vi "Set Start Trigger (Value Change).vi"(5 "Retriggerable (F)":bool, 7 "Pre-Trigger Duration (0 s)":dbl, 8 "error in (no error)":errorcluster, 9 "Trigger Channel":string, 10 "Deadband":dbl, 11 "Data Logging Specification Ref in":T1) -> (0 "error out":errorcluster, 3 "Data Logging Specification Ref out":T1)   [LabVIEW 2020, in "NI_VS Data Logging API.lvlib"]
doc: "Specifies a trigger condition on which to start logging data. You also can specify whether to log channel data immediately preceding the trigger condition and whether logging is retriggerable, meaning the data logging session watches for subsequent occurrences of the start trigger after the first logging operation finishes. By default, logging stops after one operation.\n\nYou must manually select the polymorphic instance to use."
uses:
  <vilib>/NI VeriStand/Execution/DataLogging/NI_VS Data Logging API.lvlib
  <vilib>/NI VeriStand/Execution/DataLogging/DataLoggingSpecification Ref.ctl
  NationalInstruments.VeriStand.ClientAPI
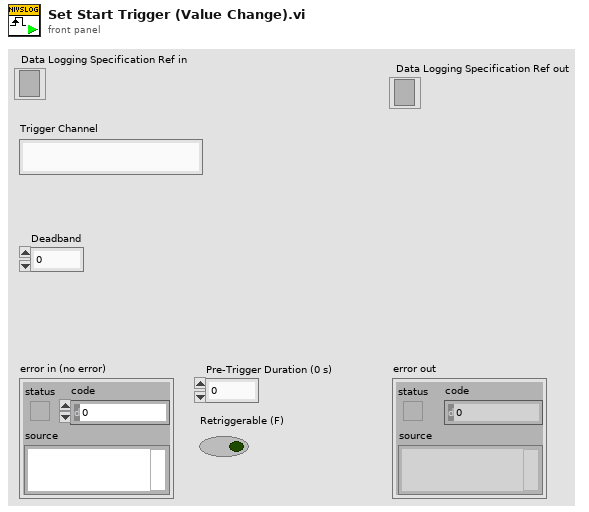
[diagram p1: front panel]
types:
  T1 = typedef "NI_VS Data Logging API.lvlib/DataLoggingSpecification Ref.ctl" = refnum<k24>
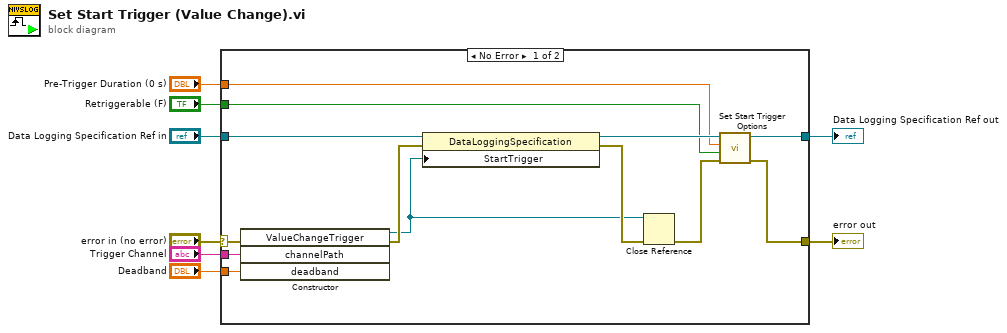
[diagram p0: block diagram]
diagram:
  n1 = case shown="No Error" "error in (no error)" {
    selector: "error in (no error)" -> [w14 w23]
    tunnel: "Trigger Channel" -> [w13 _]
    tunnel: "Data Logging Specification Ref in" -> [w19 w22]
    tunnel: [w16 w22] -> w6
    tunnel: [w15 w23] -> w5
    tunnel: "Deadband" -> [w11 _]
    tunnel: "Retriggerable (F)" -> [w10 _]
    tunnel: "Pre-Trigger Duration (0 s)" -> [w9 _]
    frame No Error {
      n2 = constructor class="ValueChangeTrigger"(error in=w14, "channelPath"=w13, "deadband"=w11) -> (reference out=w12:refnum<k24>, error out=w21:errorcluster)  [unwired: 2 in, 3 out]
      n3 = property class="DataLoggingSpecification"(reference=w19, error in=w21, "StartTrigger"=w12) -> (reference out=w18:T1, error out=w20:errorcluster)
      n4 = Close Reference(reference=w12, error in (no error)=w20) -> (error out=w17:errorcluster)
      n5 = call <vilib>:"Set Start Trigger Options.vi"("error in (no error)"=w17, "Retriggerable"=w10, "Pre-Trigger Duration"=w9, "Data Logging Specification Ref in"=w18) -> ("error out"=w15:errorcluster, "Data Logging Specification Ref out"=w16:T1)  [unwired: 6 in]
    }
    frame Error {
    }
  }
  "error out" <- w5
  "Data Logging Specification Ref out" <- w6
